vi "RC_CHANNELS_OVERRIDE_OLD.vi"(11 "Payload":T1) -> ()   [LabVIEW 2014]
uses:
  Controls/FGV Methods.ctl
panel:
  out "output packet":u8[](array[numeric]) format="%x"
  out "chan3_raw":u16
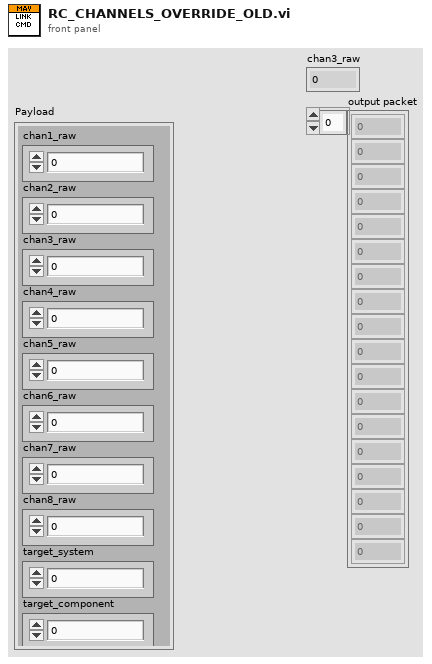
[diagram p1: front panel]
types:
  T1 = cluster{"chan1_raw":u16, "chan2_raw":u16, "chan3_raw":u16, "chan4_raw":u16, "chan5_raw":u16, "chan6_raw":u16, "chan7_raw":u16, "chan8_raw":u16, "target_system":u8, "target_component":u8}
  T2 = typedef "FGV Methods.ctl" = enum16{"Get", "Set"}
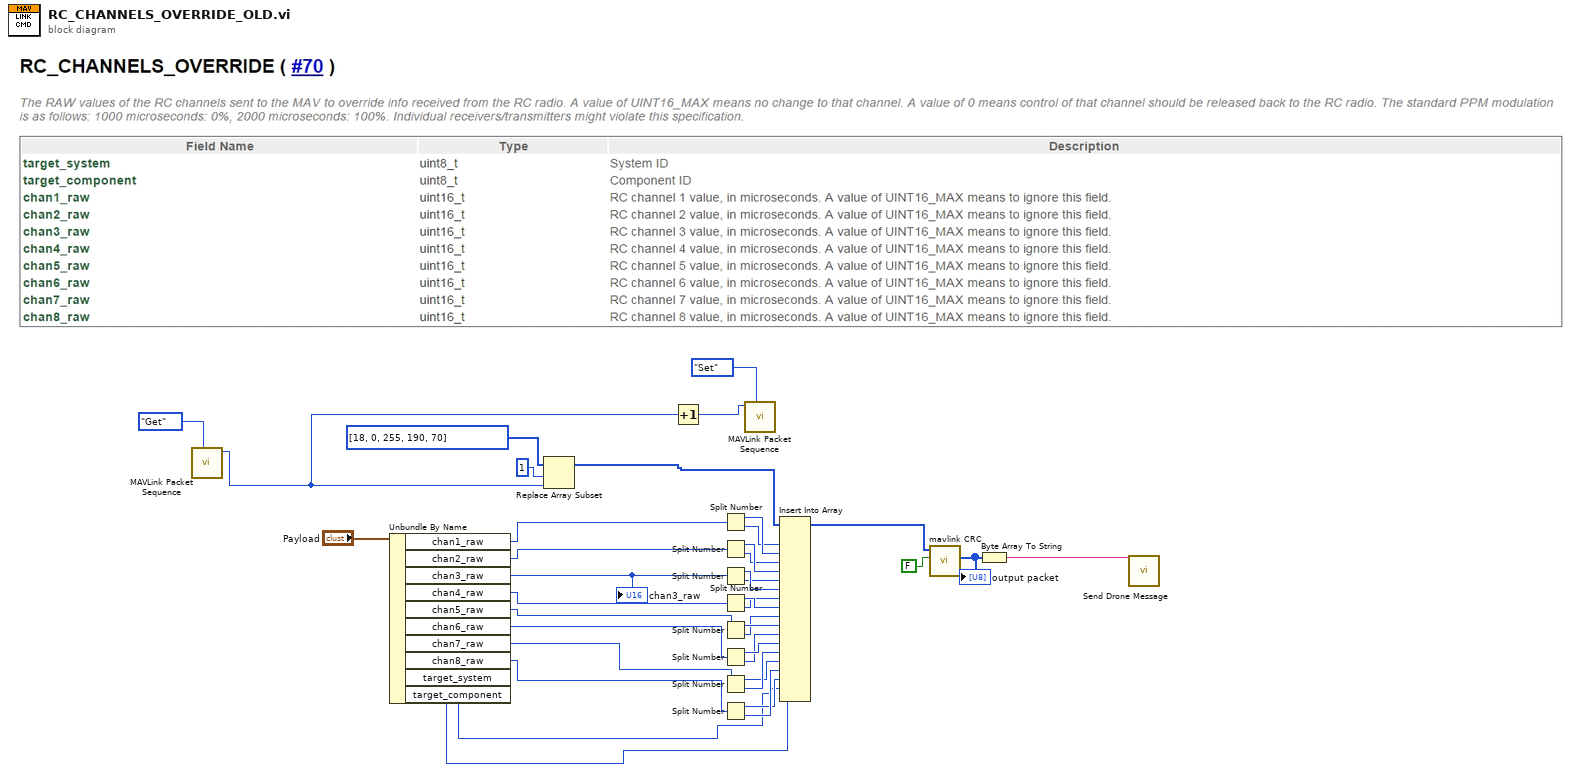
[diagram p0: block diagram]
diagram:
  n1 = call "MAVLink Packet Sequence.vi"("FGV Method"=FGV_Methods."Get") -> ("Packet Sequence Out"=w5:u8)  [unwired: 10 in]
  n2 = Unbundle By Name("Payload") -> ("chan1_raw"=w36:u16, "chan2_raw"=w33:u16, "chan3_raw"=w30:u16, "chan4_raw"=w27:u16, "chan5_raw"=w24:u16, "chan6_raw"=w21:u16, "chan7_raw"=w17:u16, "chan8_raw"=w14:u16, "target_system"=w13:u8, "target_component"=w12:u8)
  "chan3_raw" <- w30
  n3 = Replace Array Subset(array=u8[] [18, 0, 255, 190, 70], new element=w5, index=1) -> (w9:u8[])
  n4 = Increment(x=w5) -> (x+1=w6:u8)
  n5 = Split Number(x=w36) -> (hi(x)=w38:u8, lo(x)=w35:u8)
  n6 = Split Number(x=w33) -> (hi(x)=w34:u8, lo(x)=w32:u8)
  n7 = Split Number(x=w30) -> (hi(x)=w31:u8, lo(x)=w29:u8)
  n8 = Split Number(x=w27) -> (hi(x)=w28:u8, lo(x)=w26:u8)
  n9 = Split Number(x=w24) -> (hi(x)=w25:u8, lo(x)=w23:u8)
  n10 = Split Number(x=w21) -> (hi(x)=w22:u8, lo(x)=w20:u8)
  n11 = Split Number(x=w17) -> (hi(x)=w18:u8, lo(x)=w19:u8)
  n12 = Split Number(x=w14) -> (hi(x)=w15:u8, lo(x)=w16:u8)
  n13 = call "MAVLink Packet Sequence.vi"("FGV Method"=FGV_Methods."Set", "Packet Sequence In"=w6) -> ()  [unwired: 9 in, 1 out]
  n14 = Insert Into Array(array=w9, new element #1=w35, new element #2=w38, new element #3=w32, new element #4=w34, new element #5=w29, new element #6=w31, new element #7=w26, new element #8=w28, new element #9=w23, new element #10=w25, new element #11=w20, new element #12=w22, new element #13=w19, new element #14=w18, new element #15=w16, new element #16=w15, new element #17=w13, new element #18=w12) -> (w2:u8[])  [unwired: 1 in]
  n15 = call "mavlink CRC.vi"("Check (T)/ Generate (F)"=FALSE ("Check / Generate"), "byte array input"=w2) -> ("output packet"=w3:u8[])  [unwired: 8 in, 1 out]
  "output packet" <- w3
  n16 = Byte Array To String(unsigned byte array=w3) -> (string=w1:string)
  n17 = call "Send Drone Message.vi"("Message"=w1) -> ()  [unwired: 11 in]
